vi "add_to_list.vi"(8 "error in (no error)":errorcluster, 10 "String":string, 11 "StringList in":refnum<class "StringList.lvclass">) -> (0 "error out":errorcluster, 3 "StringList out":refnum<class "StringList.lvclass">)   [LabVIEW 2015, in "StringList.lvlib" / "StringList.lvclass"]
uses:
  StringList.lvclass
  StringList.lvclass/StringList.ctl
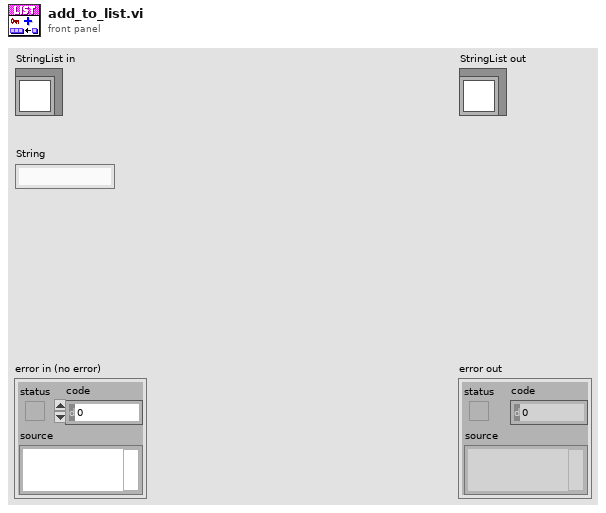
[diagram p1: front panel]
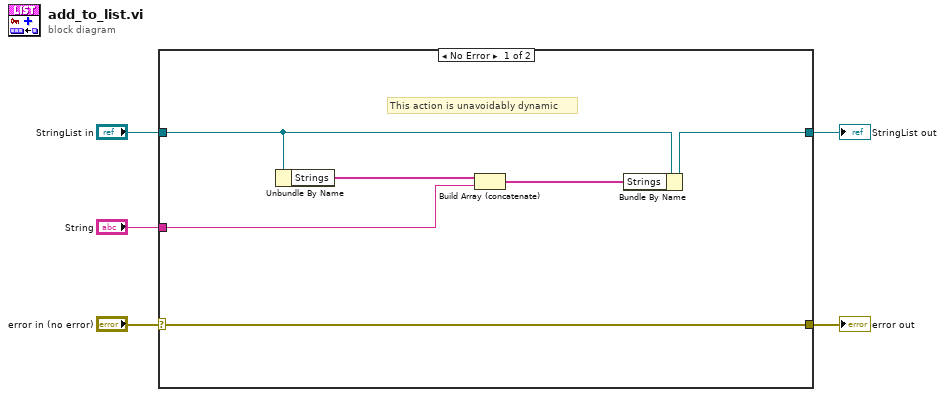
[diagram p0: block diagram]
diagram:
  n1 = case shown="No Error" "error in (no error)" {
    selector: "error in (no error)" -> [w11 w13]
    tunnel: [w11 w13] -> w4
    tunnel: [w7 w12] -> w2
    tunnel: "StringList in" -> [w10 w12]
    tunnel: "String" -> [w8 _]
    frame No Error {
      # "This action is unavoidably dynamic"
      n2 = Unbundle By Name(w10) -> ("Strings"=w9:string[])
      n3 = Build Array (concatenate)(w9, w8) -> (w6:string[])
      n4 = Bundle By Name(cluster=w10, "Strings"=w6) -> (w7:refnum<class "StringList.lvclass">)
    }
    frame Error {
    }
  }
  "error out" <- w4
  "StringList out" <- w2
